vi "Get Lockin Parameters.vi"(8 "error in (no error)":errorcluster, 11 "RP Instrument in":refnum<class "RP Instrument.lvclass">) -> (0 "error out":errorcluster, 2 "Lockin parameters":T1={"Frequency"=0.0, "Phase"=0.0, "Syncronous"=FALSE, "Points per sine wave"=0, "DDS"=FALSE, "Frequency word"=0, "Phase word"=0, "DDS modulus"=15120, "DDS clock"=125000000.0} {"DDS clock" format="%_17pHz"; "DDS modulus" format="0x%x (%d)"; "Phase" format="%#_gdeg"; "Frequency" format="%_17pHz"}, 3 "RP Instrument out":refnum<class "RP Instrument.lvclass">)   [LabVIEW 2016, in "RP Instrument.lvclass"]
uses:
  RP Instrument.lvclass
  SoftwareLockin/Lockin Parameters.ctl
  RP Status Offsets.ctl
  RP Instrument.lvclass/RP Instrument.ctl
  RP Communicator/RP Communicator.lvclass
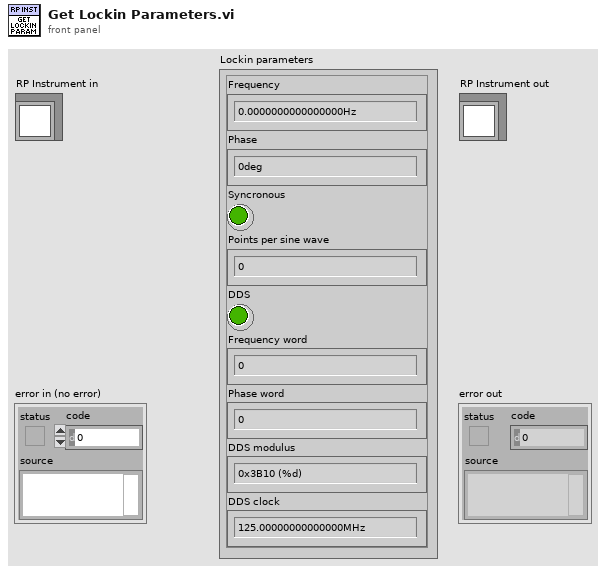
[diagram p1: front panel]
types:
  T1 = typedef "Lockin Parameters.ctl" = cluster{"Frequency":dbl, "Phase":dbl, "Syncronous":bool, "Points per sine wave":i32, "DDS":bool, "Frequency word":u32, "Phase word":u32, "DDS modulus":i64, "DDS clock":dbl}
  T2 = typedef "RP Status Offsets.ctl" = u16
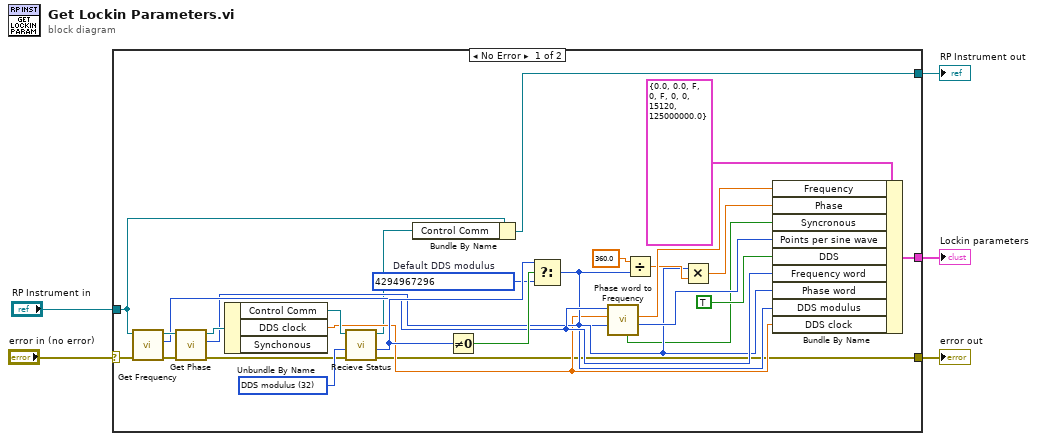
[diagram p0: block diagram]
diagram:
  n1 = case shown="No Error" "error in (no error)" {
    selector: "error in (no error)" -> [w8 w34]
    tunnel: [w7 w34] -> w4
    tunnel: [w10 w33] -> w2
    tunnel: "RP Instrument in" -> [w20 w33]
    tunnel: [w17 _] -> w1
    frame No Error {
      w28 = i64 4294967296  # Default DDS modulus
      w32 = T2 32 items=["Writer address"=0, "Record start position"=4, "Trig state and ID"=8, "Phase"=12, "X1"=16, "Y1"=20, "RxFIFO counter or  X2"=24, "TxFIFO counter or Y2"=28, "DDS modulus"=32] ("Status offsets")
      n2 = call-dynamic "Get Frequency.vi"("error in (no error)"=w8, "RP Instrument in"=w20) -> ("error out"=w27:errorcluster, "Frequency"=w14:u32, "RP Instrument out"=w26:refnum<class "RP Instrument.lvclass">)  [unwired: 7 in]
      n3 = call-dynamic "Get Phase.vi"("error in (no error)"=w27, "RP Instrument in"=w26) -> ("error out"=w25:errorcluster, "Phase"=w13:u32, "RP Instrument out"=w19:refnum<class "RP Instrument.lvclass">)  [unwired: 7 in]
      n4 = Unbundle By Name(w19) -> ("Control Comm"=w31:refnum<class "RP Communicator.lvclass">, "DDS clock"=w11:dbl)  [unwired: 1 out]
      n5 = call-dynamic "Recieve Status.vi"("error in (no error)"=w25, "Status offset"=w32, "RP Communicator in"=w31) -> ("error out"=w7:errorcluster, "Status response"=w29:u32, "RP Communicator out"=w9:refnum<class "RP Communicator.lvclass">)  [unwired: 6 in]
      n6 = Bundle By Name(cluster=w20, "Control Comm"=w9) -> (w10:refnum<class "RP Instrument.lvclass">)
      n7 = Not Equal To 0?(x=w29) -> (x != 0?=w30:bool)
      n8 = Select(t=w29, s=w30, f=w28) -> (s? t:f=w12:i64)
      n9 = call "Phase word to Frequency.vi"("DDS modulus"=w12, "DDS clock"=w11, "Phase word"=w14) -> ("Points per sine wave"=w16:u64, "Actual frequency"=w23:dbl, "Syncronous"=w6:bool)  [unwired: 6 in]
      n10 = Divide(x=360.0, y=w12) -> (x/y=w21:dbl)
      n11 = Multiply(x=w13, y=w21) -> (x*y=w18:dbl)
      n12 = Bundle By Name(cluster=T1 {"Frequency"=0.0, "Phase"=0.0, "Syncronous"=FALSE, "Points per sine wave"=0, "DDS"=FALSE, "Frequency word"=0, "Phase word"=0, "DDS modulus"=15120, "DDS clock"=125000000.0} ("Lockin parameters"), "Frequency"=w23, "Phase"=w18, "Syncronous"=w6, "Points per sine wave"=w16, "DDS"=TRUE, "Frequency word"=w14, "Phase word"=w13, "DDS modulus"=w12, "DDS clock"=w11) -> (w17:T1)
    }
    frame Error {
    }
  }
  "error out" <- w4
  "RP Instrument out" <- w2
  "Lockin parameters" <- w1
